vi "TestDriveEncoders.vi"(2 "WheelDiameter(in)":dbl=4.0, 3 "CountsPerRevolution":i32=4096, 4 "ZeroSensors":bool, 5 "RobotDriveMotors":T4[](array[typedef])) -> (0 "Drive Encoder Outputs":T3, 1 "Drive Encoder Outputs Raw":T1)   [LabVIEW 2017]
uses:
  <vilib>/Rock Robotics/WPI/MotorControl/WPI_MotorControlDeviceRef.ctl
  <vilib>/Rock Robotics/WPI/MotorControl/WPI_MotorControlType.ctl
  <vilib>/Rock Robotics/SystemInterfaces/DIO/FPGA_DIOPWMChannel.ctl
  <vilib>/Rock Robotics/WPI/PWM/WPI_PWMDeadband.ctl
  <vilib>/Rock Robotics/SystemInterfaces/DIO/FPGA_DIOChannel.ctl
  ArgosLib/Drive/MotorControl/TypeDefs/RobotDriveMotorSelectorEnum.ctl
  <vilib>/Rock Robotics/WPI/ThirdParty/Phoenix-LabVIEW/Motor Controller/Get/CTRE_Phoenix_MotorController_GetSelectedSensorData.vi
  ArgosLib/ArgosLib.lvlib
panel:
  out "Other Encoder Outputs":T2
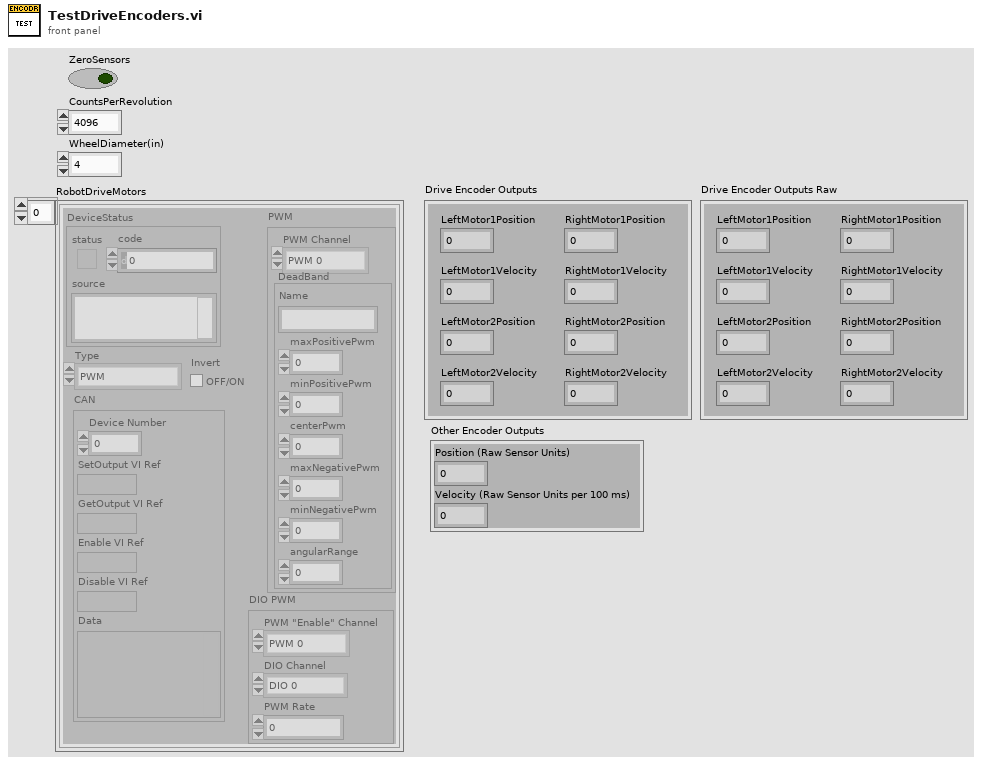
[diagram p1: front panel]
types:
  T1 = cluster{"LeftMotor1Position ":i32, "LeftMotor1Velocity":i32, "RightMotor1Velocity ":i32, "RightMotor1Position ":i32, "LeftMotor2Position ":i32, "LeftMotor2Velocity ":i32, "RightMotor2Position":i32, "RightMotor2Velocity":i32}
  T2 = cluster{"Position (Raw Sensor Units)":i32, "Velocity (Raw Sensor Units per 100 ms)":i32}
  T3 = cluster{"LeftMotor1Position ":dbl, "LeftMotor1Velocity":dbl, "RightMotor1Velocity ":dbl, "RightMotor1Position ":dbl, "LeftMotor2Position ":dbl, "LeftMotor2Velocity ":dbl, "RightMotor2Position":dbl, "RightMotor2Velocity":dbl}
  T4 = typedef "WPI_MotorControlDeviceRef.ctl" = cluster{"DeviceStatus":errorcluster, "Type":T5, "PWM":cluster{"PWM Channel":T6, "DeadBand":T7}, "CAN":cluster{"Device Number":u8, "SetOutput VI Ref":variant, "GetOutput VI Ref":variant, "Enable VI Ref":variant, "Disable VI Ref":variant, "Data":variant}, "Invert":bool, "DIO PWM":cluster{"PWM \"Enable\" Channel":T6, "DIOChannel":T8, "PWM Rate":dbl}}
  T5 = typedef "WPI_MotorControlType.ctl" = enum16{"PWM", "CAN", "DIO PWM"}
  T6 = typedef "FPGA_DIOPWMChannel.ctl" = enum8{"PWM 0", "PWM 1", "PWM 2", "PWM 3", "PWM 4", "PWM 5", "PWM 6", "PWM 7", "PWM 8", "PWM 9", "PWM MXP 0", "PWM MXP 1", "PWM MXP 2", "PWM MXP 3", "PWM MXP 4", "PWM MXP 5", "PWM MXP 6", "PWM MXP 7", "PWM MXP 8", "PWM MXP 9", "Invalid"}
  T7 = typedef "WPI_PWMDeadband.ctl" = cluster{"Name":string, "maxPositivePwm":i32, "minPositivePwm":i32, "centerPwm":i32, "maxNegativePwm":i32, "minNegativePwm":i32, "angularRange":u16}
  T8 = typedef "FPGA_DIOChannel.ctl" = enum8{"DIO 0", "DIO 1", "DIO 2", "DIO 3", "DIO 4", "DIO 5", "DIO 6", "DIO 7", "DIO 8", "DIO 9", "DIO MXP 0", "DIO MXP 1", "DIO MXP 2", "DIO MXP 3", "DIO MXP 4", "DIO MXP 5", "DIO MXP 6", "DIO MXP 7", "DIO MXP 8", "DIO MXP 9", "DIO MXP 10", "DIO MXP 11", "DIO MXP 12", "DIO MXP 13", "DIO MXP 14", "DIO MXP 15", "SPI Port CS1", "SPI Port CS2", "SPI Port CS3", "SPI Port MISO", "SPI Port MOSI", "Invalid"}
  T9 = typedef "ArgosLib.lvlib/RobotDriveMotorSelectorEnum.ctl" = enum16{"Left Motor 1", "Right Motor 1", "Left Motor 2", "Right Motor 2", "Left Motor 3", "Right Motor 3"}
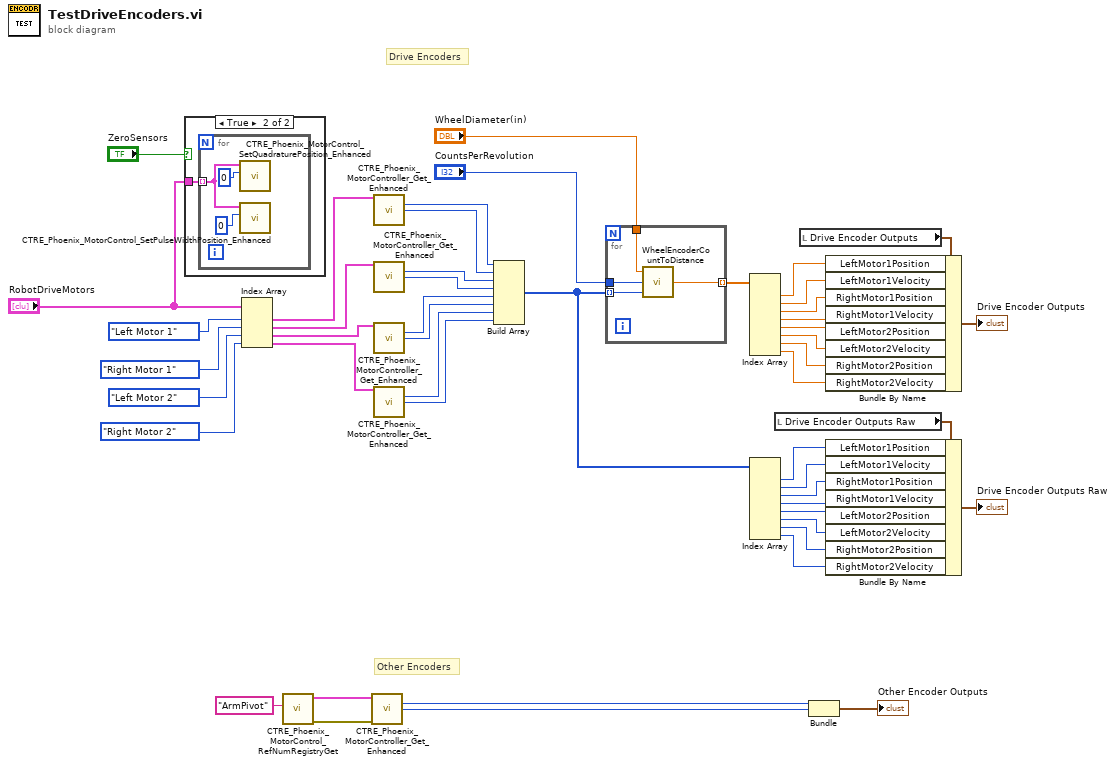
[diagram p0: block diagram]
diagram:
  # "Other Encoders"
  # "Drive Encoders"
  n1 = case shown="True" "ZeroSensors" {
    tunnel: "RobotDriveMotors" -> [_ w49]
    frame False {
    }
    frame True {
      n2 = for {
        tunnel: w49 -> [w52] mode=indexing
        n3 = call <vilib>:"CTRE_Phoenix_MotorControl_SetQuadraturePosition_Enhanced.vi"("New Position"=0, "PhoenixMotorControlDevRef"=w52) -> ()  [unwired: 8 in, 2 out]
        n4 = call <vilib>:"CTRE_Phoenix_MotorControl_SetPulseWidthPosition_Enhanced.vi"("New Position"=0, "PhoenixMotorControlDevRef"=w52) -> ()  [unwired: 8 in, 2 out]
      }
    }
  }
  n5 = Index Array(array="RobotDriveMotors", index #1=RobotDriveMotorSelectorEnum."Left Motor 1" ("Motor Selector Enum"), index #2=RobotDriveMotorSelectorEnum."Right Motor 1" ("Motor Selector Enum"), index #3=RobotDriveMotorSelectorEnum."Left Motor 2" ("Motor Selector Enum"), index #4=RobotDriveMotorSelectorEnum."Right Motor 2" ("Motor Selector Enum")) -> (element #1=w44:T4, element #2=w43:T4, element #3=w42:T4, element #4=w41:T4)
  n6 = call <vilib>:"CTRE_Phoenix_MotorControl_RefNumRegistryGet.vi"("refnum name"="ArmPivot") -> ("error out"=w17:errorcluster, "PhoenixMotorControlDevRef"=w18:T4)  [unwired: 9 in]
  n7 = call-poly <vilib>:"CTRE_Phoenix_MotorController_Get_Enhanced.vi"("PhoenixMotorControlDevRef"=w18, "error in"=w17) -> ("Position (Raw Sensor Units)"=w16:i32, "Velocity (Raw Sensor Units per 100 ms)"=w15:i32)  [unwired: 10 in, 2 out]
  n8 = call-poly <vilib>:"CTRE_Phoenix_MotorController_Get_Enhanced.vi"("PhoenixMotorControlDevRef"=w44) -> ("Position (Raw Sensor Units)"=w40:i32, "Velocity (Raw Sensor Units per 100 ms)"=w39:i32)  [unwired: 11 in, 2 out]
  n9 = call-poly <vilib>:"CTRE_Phoenix_MotorController_Get_Enhanced.vi"("PhoenixMotorControlDevRef"=w43) -> ("Position (Raw Sensor Units)"=w34:i32, "Velocity (Raw Sensor Units per 100 ms)"=w33:i32)  [unwired: 11 in, 2 out]
  n10 = call-poly <vilib>:"CTRE_Phoenix_MotorController_Get_Enhanced.vi"("PhoenixMotorControlDevRef"=w42) -> ("Position (Raw Sensor Units)"=w38:i32, "Velocity (Raw Sensor Units per 100 ms)"=w37:i32)  [unwired: 11 in, 2 out]
  n11 = call-poly <vilib>:"CTRE_Phoenix_MotorController_Get_Enhanced.vi"("PhoenixMotorControlDevRef"=w41) -> ("Position (Raw Sensor Units)"=w36:i32, "Velocity (Raw Sensor Units per 100 ms)"=w35:i32)  [unwired: 11 in, 2 out]
  n12 = Build Array(w40, w39, w34, w33, w38, w37, w36, w35) -> (w2:i32[])
  n13 = for {
    tunnel: w2 -> [w56] mode=indexing
    tunnel: [w55] -> w32 mode=indexing
    tunnel: "CountsPerRevolution" -> [w54]
    tunnel: "WheelDiameter(in)" -> [w53]
    n14 = call "WheelEncoderCountToDistance.vi"("EncoderCounts"=w56, "CountsPerRevolution"=w54, "WheelDiameter(in)"=w53) -> ("Output(in)"=w55:dbl)
  }
  n15 = Index Array(array=w32) -> (element #1=w26:dbl, element #2=w25:dbl, element #3=w24:dbl, element #4=w23:dbl, element #5=w22:dbl, element #6=w21:dbl, element #7=w20:dbl, element #8=w19:dbl)  [unwired: 8 in]
  n16 = Index Array(array=w2) -> (element #1=w3:i32, element #2=w4:i32, element #3=w5:i32, element #4=w6:i32, element #5=w7:i32, element #6=w8:i32, element #7=w9:i32, element #8=w10:i32)  [unwired: 8 in]
  n17 = local read "Drive Encoder Outputs Raw"() -> (w11:T1)
  n18 = local read "Drive Encoder Outputs"() -> (w12:T3)
  n19 = Bundle("Position (Raw Sensor Units)"=w16, "Velocity (Raw Sensor Units per 100 ms)"=w15) -> (→"Other Encoder Outputs":T2)  [unwired: 1 in]
  n20 = Bundle By Name(cluster=w12, "LeftMotor1Position"=w26, "LeftMotor1Velocity"=w25, "RightMotor1Position"=w24, "RightMotor1Velocity"=w23, "LeftMotor2Position"=w22, "LeftMotor2Velocity"=w21, "RightMotor2Position"=w20, "RightMotor2Velocity"=w19) -> (→"Drive Encoder Outputs":T3)
  n21 = Bundle By Name(cluster=w11, "LeftMotor1Position"=w3, "LeftMotor1Velocity"=w4, "RightMotor1Position"=w5, "RightMotor1Velocity"=w6, "LeftMotor2Position"=w7, "LeftMotor2Velocity"=w8, "RightMotor2Position"=w9, "RightMotor2Velocity"=w10) -> (→"Drive Encoder Outputs Raw":T1)
